vi "Write library name.vi"(8 "error in":errorcluster, 10 "library name":string, 11 "editorscriptingobject in":refnum<class "editorscriptingobject.lvclass">) -> (0 "error out":errorcluster, 3 "editorscriptingobject out":refnum<class "editorscriptingobject.lvclass">)   [LabVIEW 2013, in "editorscriptingobject.lvclass"]
uses:
  editorscriptingobject.lvclass
  editorscriptingobject.lvclass/editorscriptingobject.ctl
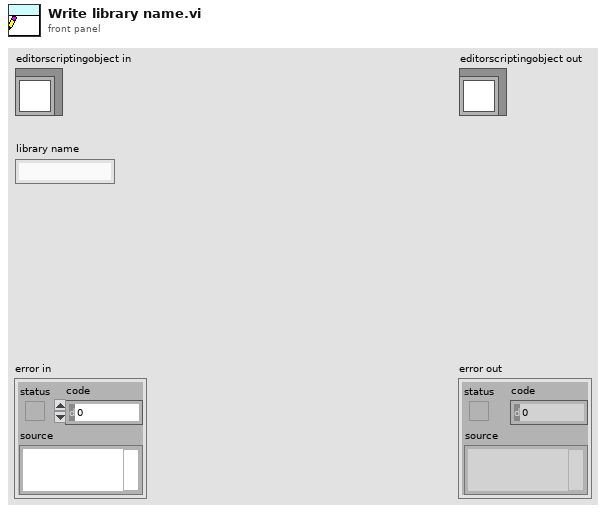
[diagram p1: front panel]
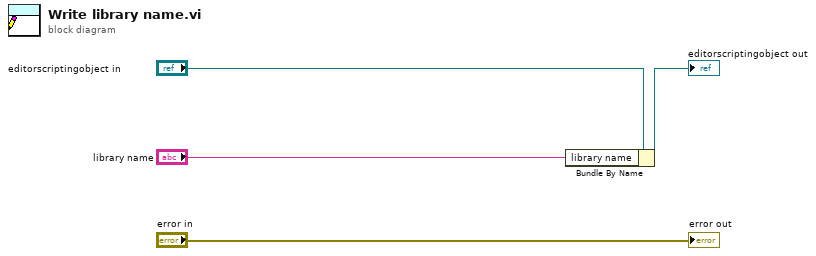
[diagram p0: block diagram]
diagram:
  n1 = Bundle By Name(cluster="editorscriptingobject in", "library name"="library name") -> (→"editorscriptingobject out":refnum<class "editorscriptingobject.lvclass">)
  "error out" <- "error in"
